vi "T chart calculations.vi"(0 "Scale Control":T8, 2 "clear chart":bool, 7 "WaveformChart in":refnum<vi>, 11 "T cont":T1={"T exec"={"T mode"=enum."Exit", "exec setpoint"=30.0, "reset"=FALSE, "man power"=0.5, "man"=FALSE, "log"=FALSE, "clear"=FALSE}, "T status"={"Control status"=enum."Below Control Band", "Temp"=0.0, "Power"=0.0, "Time in settle band"=0.0, "Settled"=FALSE, "Low"=FALSE, "High"=FALSE, "Setpoint"=30.0, "Control"=FALSE, "In Settle Band"=FALSE}, "T params"={"Setpoint"=50.0, "Control Bandwidth"=4.0, "Integral Time"=30.0, "Int\nON"=TRUE, "Derivative Tme"=0.5, "Der\nON"=TRUE, "Settle Bandwidth"=1.0, "Settle Time"=60.0}, "utility"={"meas index"=300, "wait (ms)"=0, "H Vmax"=8.5, "power out"=0.0, "heat volt out"=0.0, "heat volt in"=0.0, "therm volt"=0.0, "t T P hist"=[], "cont hist"=[]}} {"utility"."therm volt" format="%_6g"; "utility"."heat volt in" format="%_6g"; "utility"."heat volt out" format="%_6g"; "utility"."power out" format="%_6g"; "utility"."H Vmax" format="%_6g"; "T exec"."man power" format="%_6g"; "T exec"."exec setpoint" format="%_6g"; "T params"."Settle Time" step=1.0; "T params"."Settle Bandwidth" step=0.01; "T params"."Derivative Tme" step=0.01; "T params"."Integral Time" step=1.0; "T params"."Control Bandwidth" step=0.1; "T params"."Setpoint" step=0.1; "T status"."Setpoint" format="%_6g"; "T status"."Power" format="%_6g"; "T status"."Temp" format="%_6g"}) -> (4 "T chart cluster":T9, 15 "Setpoint":dbl)   [LabVIEW 2019]
doc: "This is a Bug C(T) subVI.\n\nThis subVI handles the scale change requests for the temeperature chart, and does the calulations for the temperature chart in the bug experiment.\n\nIt scales the power varaible to be normalized to [0,1] on the vertical temp scale dynamicallly. It clears the power history on scale change.\n\nIt also clears the chart on command.\n\nPaul K Dixon\nP3600\nCSUSB Physics"
uses:
  typedefs/scale control.ctl
  typedefs/temp cont cluster.ctl
  typedefs/temp exec cluster.ctl
  typedefs/temp mode enum.ctl
  typedefs/temp indicator.ctl
  typedefs/temp control status.ctl
  typedefs/PID control parameters.ctl
  typedefs/temp cont utility.ctl
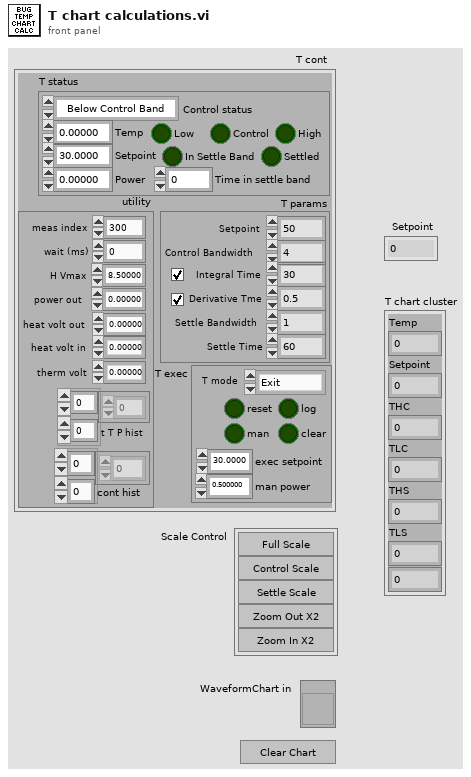
[diagram p1: front panel]
types:
  T1 = typedef "temp cont cluster.ctl" = cluster{"T exec":T2, "T status":T4, "T params":T6, "utility":T7}
  T2 = typedef "temp exec cluster.ctl" = cluster{"T mode":T3, "exec setpoint":dbl, "reset":bool, "man power":dbl, "man":bool, "log":bool, "clear":bool}
  T3 = typedef "temp mode enum.ctl" = enum16{"settling", "measuring", "holding", "Exit"}
  T4 = typedef "temp indicator.ctl" = cluster{"Control status":T5, "Temp":dbl, "Power":dbl, "Time in settle band":dbl, "Settled":bool, "Low":bool, "High":bool, "Setpoint":dbl, "Control":bool, "In Settle Band":bool}
  T5 = typedef "temp control status.ctl" = enum16{"In Settle Band", "In Control Band", "Below Control Band", "Above Control Band"}
  T6 = typedef "PID control parameters.ctl" = cluster{"Setpoint":dbl, "Control Bandwidth":dbl, "Integral Time":dbl, "Int\nON":bool, "Derivative Tme":dbl, "Der\nON":bool, "Settle Bandwidth":dbl, "Settle Time":dbl}
  T7 = typedef "temp cont utility.ctl" = cluster{"meas index":i32, "wait (ms)":i32, "H Vmax":dbl, "power out":dbl, "heat volt out":dbl, "heat volt in":dbl, "therm volt":dbl, "t T P hist":dbl[][], "cont hist":dbl[][]}
  T8 = typedef "scale control.ctl" = cluster{"Full Scale":bool, "Control Scale":bool, "Settle Scale":bool, "Zoom Out X2":bool, "Zoom In X2":bool}
  T9 = cluster{"Temp":dbl, "Setpoint":dbl, "THC":dbl, "TLC":dbl, "THS":dbl, "TLS":dbl, dbl}
  T10 = cluster{"temp out":dbl, dbl, dbl, dbl, dbl, dbl, dbl}[]
  T11 = cluster{"temp out":dbl, dbl, dbl, dbl, dbl, dbl, dbl}
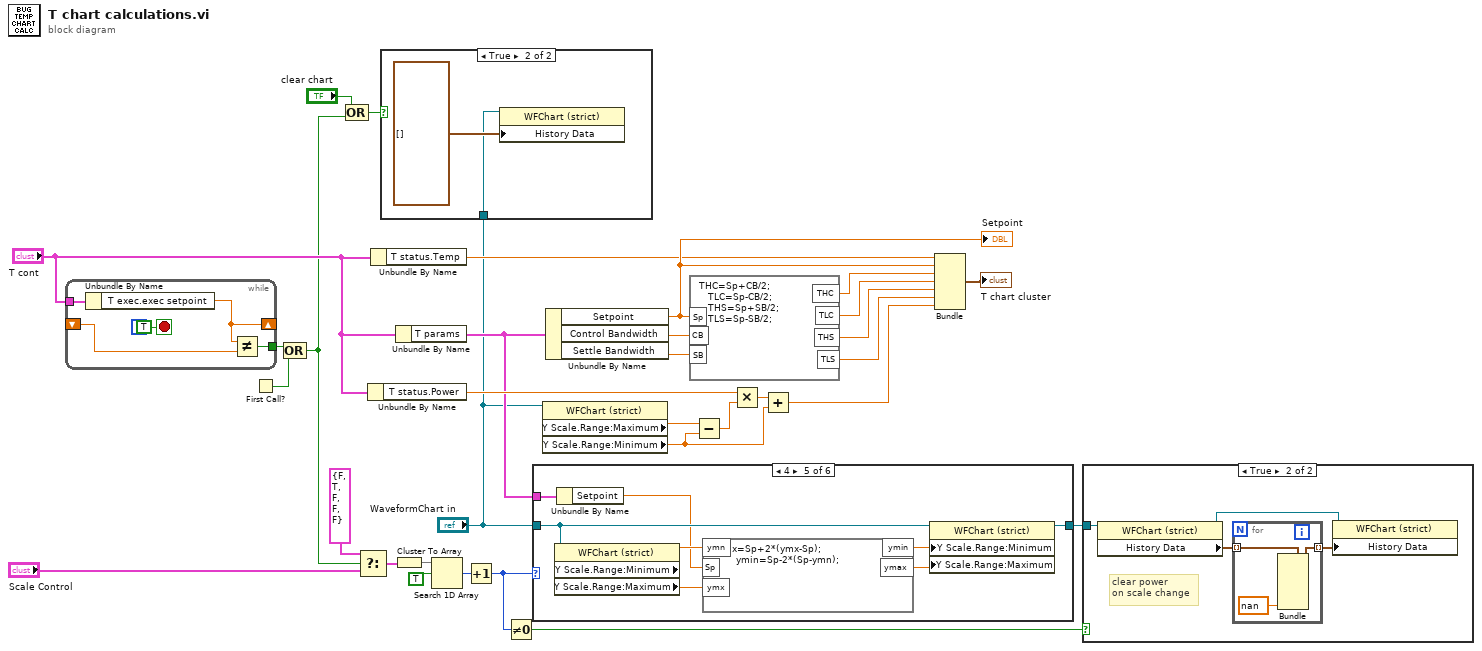
[diagram p0: block diagram]
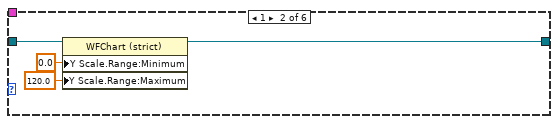
[diagram p5: hidden frame]
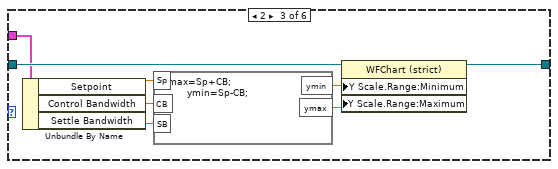
[diagram p6: hidden frame]
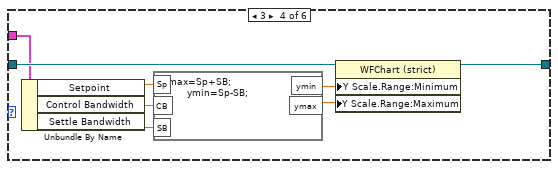
[diagram p7: hidden frame]
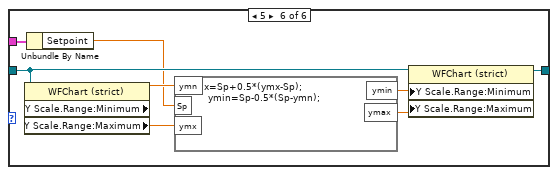
[diagram p8: hidden frame]
diagram:
  n1 = while {
    tunnel: "T cont" -> [w37]
    shift-right: [w35] -> _
    shift-left: _ -> [w36]
    tunnel: [w33] -> w2
    stop <- TRUE stop-if-true
    n2 = Unbundle By Name(w37) -> ("T exec.exec setpoint"=w35:dbl)
    n3 = Not Equal?(x=w35, y=w36) -> (x != y?=w33:bool)
  }
  n4 = First Call?() -> (First Call?: T/F=w1:bool)
  n5 = Compound Arithmetic op=OR(w2, w1) -> (w3:bool)
  n6 = Compound Arithmetic op=OR("clear chart", w3) -> (w6:bool)
  n7 = Select(t=T8 {"Full Scale"=FALSE, "Control Scale"=TRUE, "Settle Scale"=FALSE, "Zoom Out X2"=FALSE, "Zoom In X2"=FALSE} ("Scale Control"), s=w3, f="Scale Control") -> (s? t:f=w9:T8)
  n8 = Unbundle By Name("T cont") -> ("T status.Power"=w13:dbl)
  n9 = Unbundle By Name("T cont") -> ("T status.Temp"=w11:dbl)
  n10 = case shown="True" w6 {
    tunnel: "WaveformChart in" -> [_ w38]
    frame False {
    }
    frame True {
      n11 = property on="Property Node" class="WFChart (strict)"(reference=w38, "History Data"=T10 []) -> ()  [unwired: 1 in, 2 out]
    }
  }
  n12 = Cluster To Array(cluster=w9) -> (array=w16:bool[])
  n13 = Unbundle By Name("T cont") -> ("T params"=w12:T6)
  n14 = Search 1D Array(1D array=w16, element=TRUE) -> (index of element=w14:i32)  [unwired: 1 out]
  n15 = Increment(x=w14) -> (x+1=w31:i32)
  n16 = Not Equal To 0?(x=w31) -> (x != 0?=w32:bool)
  n17 = case shown="4" w31 {
    tunnel: w12 -> [_ _ w48 w56 w62 w70]
    tunnel: "WaveformChart in" -> [w40 w42 w50 w58 w64 w71]
    tunnel: [w40 w41 w49 w57 w63 w72] -> w30
    frame 0, Default {
    }
    frame 1 {
      n18 = property on="Property Node" class="WFChart (strict)"(reference=w42, "Y Scale.Range:Minimum"=0.0, "Y Scale.Range:Maximum"=120.0) -> (reference out=w41:refnum<vi>)  [unwired: 1 in, 1 out]
    }
    frame 2 {
      n19 = Unbundle By Name(w48) -> ("Setpoint"=w47:dbl, "Control Bandwidth"=w46:dbl, "Settle Bandwidth"=w45:dbl)
      n20 = formula code="ymax=Sp+CB;\n        ymin=Sp-CB;"("Sp"=w47, "CB"=w46, "SB"=w45) -> ("ymax"=w51:dbl, "ymin"=w52:dbl)
      n21 = property on="Property Node" class="WFChart (strict)"(reference=w50, "Y Scale.Range:Minimum"=w52, "Y Scale.Range:Maximum"=w51) -> (reference out=w49:refnum<vi>)  [unwired: 1 in, 1 out]
    }
    frame 3 {
      n22 = Unbundle By Name(w56) -> ("Setpoint"=w55:dbl, "Control Bandwidth"=w54:dbl, "Settle Bandwidth"=w53:dbl)
      n23 = formula code="ymax=Sp+SB;\n        ymin=Sp-SB;"("Sp"=w55, "CB"=w54, "SB"=w53) -> ("ymax"=w59:dbl, "ymin"=w60:dbl)
      n24 = property on="Property Node" class="WFChart (strict)"(reference=w58, "Y Scale.Range:Minimum"=w60, "Y Scale.Range:Maximum"=w59) -> (reference out=w57:refnum<vi>)  [unwired: 1 in, 1 out]
    }
    frame 4 {
      n25 = property on="Property Node" class="WFChart (strict)"(reference=w64) -> ("Y Scale.Range:Minimum"=w66:dbl, "Y Scale.Range:Maximum"=w65:dbl)  [unwired: 1 in, 2 out]
      n26 = Unbundle By Name(w62) -> ("Setpoint"=w61:dbl)
      n27 = formula code="ymax=Sp+2*(ymx-Sp);\n        ymin=Sp-2*(Sp-ymn);"("ymn"=w66, "Sp"=w61, "ymx"=w65) -> ("ymax"=w67:dbl, "ymin"=w68:dbl)
      n28 = property on="Property Node" class="WFChart (strict)"(reference=w64, "Y Scale.Range:Minimum"=w68, "Y Scale.Range:Maximum"=w67) -> (reference out=w63:refnum<vi>)  [unwired: 1 in, 1 out]
    }
    frame 5 {
      n29 = property on="Property Node" class="WFChart (strict)"(reference=w71) -> ("Y Scale.Range:Minimum"=w74:dbl, "Y Scale.Range:Maximum"=w73:dbl)  [unwired: 1 in, 2 out]
      n30 = Unbundle By Name(w70) -> ("Setpoint"=w69:dbl)
      n31 = formula code="ymax=Sp+0.5*(ymx-Sp);\n        ymin=Sp-0.5*(Sp-ymn);"("ymn"=w74, "Sp"=w69, "ymx"=w73) -> ("ymax"=w75:dbl, "ymin"=w76:dbl)
      n32 = property on="Property Node" class="WFChart (strict)"(reference=w71, "Y Scale.Range:Minimum"=w76, "Y Scale.Range:Maximum"=w75) -> (reference out=w72:refnum<vi>)  [unwired: 1 in, 1 out]
    }
  }
  n33 = property class="WFChart (strict)"(reference="WaveformChart in") -> ("Y Scale.Range:Maximum"=w20:dbl, "Y Scale.Range:Minimum"=w19:dbl)  [unwired: 1 in, 2 out]
  n34 = Unbundle By Name(w12) -> ("Setpoint"=w28:dbl, "Control Bandwidth"=w22:dbl, "Settle Bandwidth"=w21:dbl)
  "Setpoint" <- w28
  n35 = formula code="THC=Sp+CB/2;\n   TLC=Sp-CB/2;\n   THS=Sp+SB/2;\n   TLS=Sp-SB/2;"("Sp"=w28, "CB"=w22, "SB"=w21) -> ("THC"=w27:dbl, "TLC"=w25:dbl, "THS"=w26:dbl, "TLS"=w24:dbl)
  n36 = Subtract(x=w20, y=w19) -> (x-y=w17:dbl)
  n37 = Multiply(x=w13, y=w17) -> (x*y=w18:dbl)
  n38 = Add(x=w18, y=w19) -> (x+y=w23:dbl)
  n39 = Bundle("Temp"=w11, "Setpoint"=w28, "THC"=w27, "TLC"=w25, "THS"=w26, "TLS"=w24, w23) -> (→"T chart cluster":T9)  [unwired: 1 out]
  n40 = case shown="True" w32 {
    tunnel: w30 -> [_ w77]
    frame False {
    }
    frame True {
      # "clear power\non scale change"
      n41 = property class="WFChart (strict)"(reference=w77) -> (reference out=w80:refnum<vi>, "History Data"=w78:T10)  [unwired: 1 in, 1 out]
      n42 = for {
        tunnel: w78 -> [w83] mode=indexing
        tunnel: [w82] -> w79 mode=indexing
        n43 = Bundle(cluster=w83, nan) -> (w82:T11)  [unwired: 6 in]
      }
      n44 = property on="Property Node" class="WFChart (strict)"(reference=w80, "History Data"=w79) -> ()  [unwired: 1 in, 2 out]
    }
  }
